vi "Modulate symbols.vi"(7 "input bit stream":i8[](array[numeric]), 8 "error in (no error)":errorcluster, 9 "pulse shaping filter coefficients":dbl[](array[numeric]) format="%.2f", 11 "system parameters":T1 {"symbol map" format="%.3f"}) -> (0 "error out":errorcluster, 2 "symbols out":cdb[](array[numeric]) format="%.2f", 3 "output complex waveform":T2 {"Y" format="%.3f"; "dt" format="%^.2e"; "t0" format="%.4f"})   [LabVIEW 2011]
uses:
  <vilib>/addons/Modulation/Analog/controls/Complex Data Waveform.ctl
  <vilib>/addons/Modulation/niAMT.lvlib
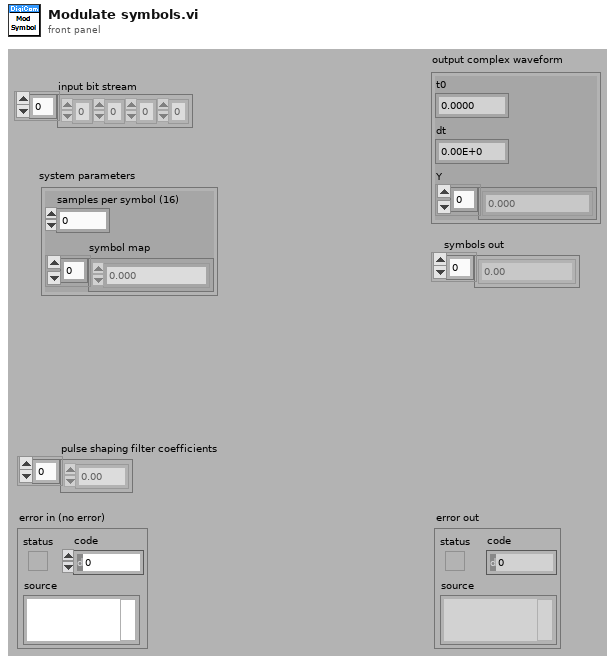
[diagram p1: front panel]
types:
  T1 = cluster{"samples per symbol (16)":i32, "symbol map":cdb[]}
  T2 = typedef "niAMT.lvlib/Complex Data Waveform.ctl" = cluster{"t0":dbl, "dt":dbl, "Y":cdb[]}
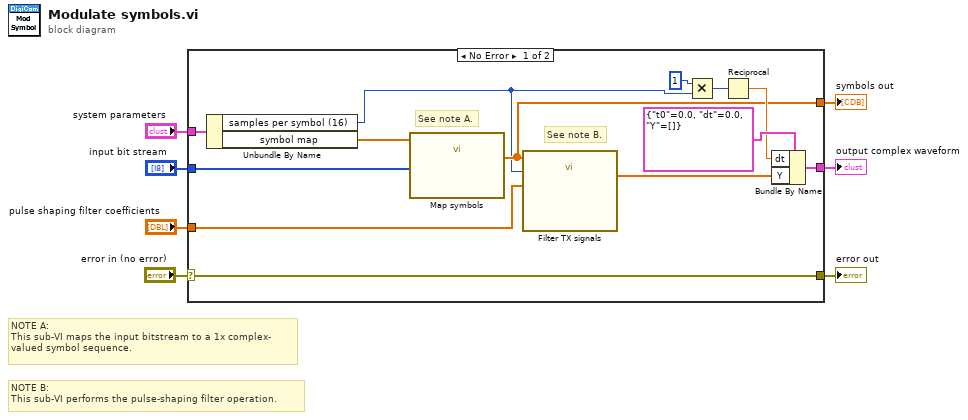
[diagram p0: block diagram]
diagram:
  # "NOTE A:\nThis sub-VI maps the input bitstream to a 1x complex-\nvalued symbol sequence."
  # "NOTE B:\nThis sub-VI performs the pulse-shaping filter operation."
  n1 = case shown="No Error" "error in (no error)" {
    selector: "error in (no error)" -> [w9 w21]
    tunnel: "system parameters" -> [w16 _]
    tunnel: "pulse shaping filter coefficients" -> [w11 _]
    tunnel: "input bit stream" -> [w14 _]
    tunnel: [w9 w21] -> w2
    tunnel: [w20 _] -> w4
    tunnel: [w13 _] -> w3
    frame No Error {
      # "See note A."
      # "See note B."
      n2 = Unbundle By Name(w16) -> ("samples per symbol (16)"=w12:i32, "symbol map"=w15:cdb[])
      n3 = call "Map symbols.vi"("Input Bit Stream"=w14, "Symbol Map"=w15) -> ("Symbols"=w13:cdb[])  [unwired: 9 in]
      n4 = call "Filter TX signals.vi"("Pulse Shaping Filter Coefficients"=w11, "Samples Per Symbol (16)"=w12, "Symbols"=w13) -> ("Filtered Samples"=w10:cdb[])  [unwired: 8 in]
      n5 = Multiply(x=1, y=w12) -> (x*y=w19:i32)
      n6 = Reciprocal(x=w19) -> (1/x=w17:dbl)
      n7 = Bundle By Name(cluster=T2 {"t0"=0.0, "dt"=0.0, "Y"=[]} ("Output Complex Waveform"), "dt"=w17, "Y"=w10) -> (w20:T2)
    }
    frame Error {
    }
  }
  "error out" <- w2
  "output complex waveform" <- w4
  "symbols out" <- w3
